vi "condAmbientalesIniciales.vi"(8 "error in (no error)":errorcluster, 11 "Equipo in":refnum<class "Equipo.lvclass">) -> (0 "error out":errorcluster, 3 "Equipo out":refnum<class "Equipo.lvclass">)   [LabVIEW 2019, in "Equipo.lvclass"]
uses:
  Equipo.lvclass
panel:
  out "humedad":dbl
  out "presion":dbl
  in  "salir":bool
  out "temperatura":dbl
  # "[°C]"
  # "[hPa]"
  # "[%]"
  # "Humedad"
  # "Presión"
  # "Temperatura"
  # "Condiciones Ambientales \nINICIALES"
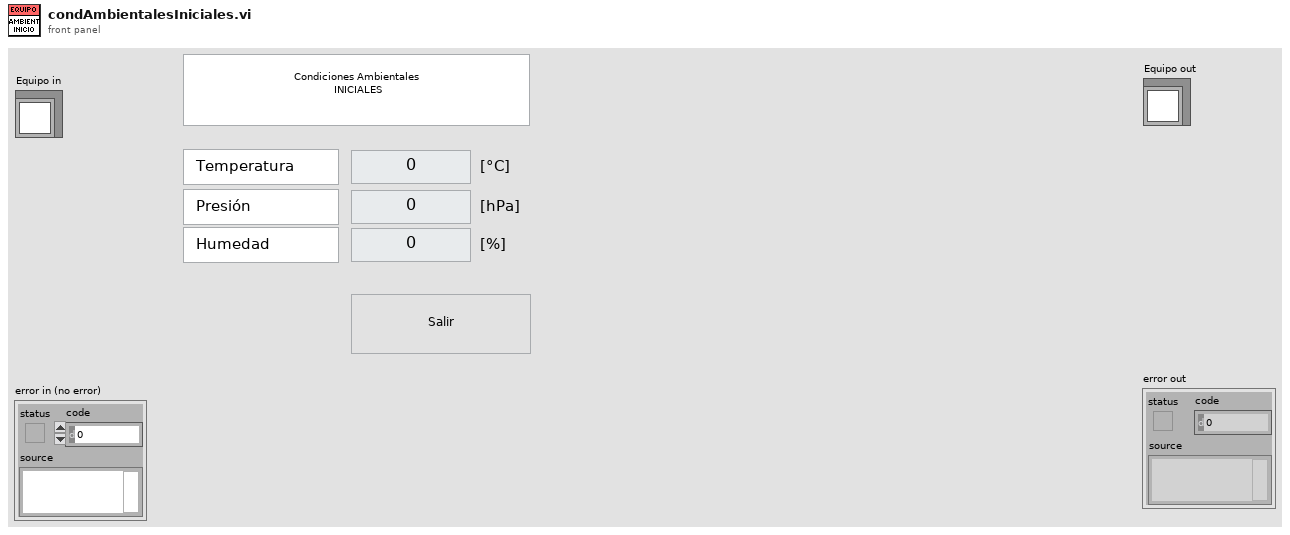
[diagram p1: front panel]
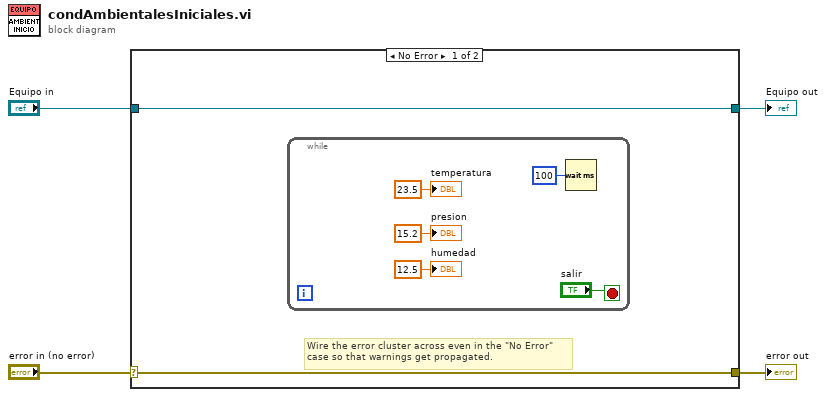
[diagram p0: block diagram]
diagram:
  n1 = case shown="No Error" "error in (no error)" {
    selector: "error in (no error)" -> [w5 w13]
    tunnel: [w5 w13] -> w3
    tunnel: [w6 w12] -> w1
    tunnel: "Equipo in" -> [w6 w12]
    frame No Error {
      # "Wire the error cluster across even in the \"No Error\"\ncase so that warnings get propagated."
      n2 = while {
        stop <- "salir" stop-if-true
        n3 = Wait (ms)(milliseconds to wait=u32 100) -> ()  [unwired: 1 out]
        "temperatura" <- 23.5 ("temperatura")
        "presion" <- 15.2 ("presion")
        "humedad" <- 12.5 ("humedad")
      }
    }
    frame Error {
    }
  }
  "error out" <- w3
  "Equipo out" <- w1
